vi "PanelUpdates.vi"(8 "error in (no error)":errorcluster, 10 "Defer Panel Updates":bool, 11 "VI in":refnum<vi>) -> (0 "error out":errorcluster)   [LabVIEW 2017, in "Shared Variables CD 2.0 Configuration.lvlib"]
uses:
  Shared Variables CD 2.0 Configuration.lvlib
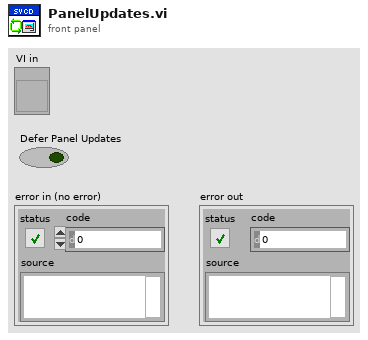
[diagram p1: front panel]
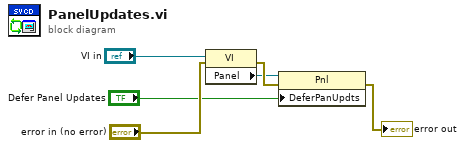
[diagram p0: block diagram]
diagram:
  n1 = property class="VI"(reference="VI in", error in="error in (no error)") -> (error out=w6:errorcluster, "Panel"=w3:refnum<vi>)  [unwired: 1 out]
  n2 = property on="Property Node" class="Pnl"(reference=w3, error in=w6, "DeferPanUpdts"="Defer Panel Updates") -> (error out=→"error out":errorcluster)  [unwired: 1 out]
